vi "FormatTableStyle.vi"(7 "Format Command":T1, 8 "Error In":errorcluster, 9 "Row Index":i32, 10 "Parameter (Optional)":i32, 11 "Table reference Array":refnum<vi>[](array[refnum])) -> (0 "Error Out":errorcluster)   [LabVIEW 2012]
doc: "SciScan 1.2 160622\nThis VI implements the formatting of table data which includes highlighting, unhighlighting, and modifying visible rows (due to scrolling).\n\n<b>INPUTS</b>\n--------\n<b>Format Command </b> - Formatting action needs to be be taken\n<b>Table references array </b>- Array containing references of the tables of interest\n<b>Row </b>- Row number that needs to be fromatted"
uses:
  FormatTableStyle_Commands.ctl
  <vilib>/Utility/miscctls.llb/LVRowAndColumnTypeDef.ctl
  <vilib>/Utility/miscctls.llb/LVRowAndColumnUnsignedTypeDef.ctl
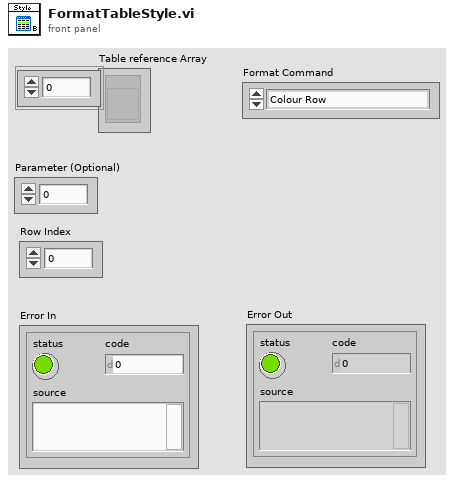
[diagram p1: front panel]
types:
  T1 = typedef "FormatTableStyle_Commands.ctl" = enum16{"Colour Row", "Uncolour Row", "Bold Row", "Clear table", "UpdateVisibleRows", "Set Row Height", "Enabled Row style", "Disabled Row Style"}
  T2 = typedef "LVRowAndColumnTypeDef.ctl" = cluster{"Row":i32, "Column":i32}
  T3 = typedef "LVRowAndColumnUnsignedTypeDef.ctl" = cluster{"Row":u32, "Column":u32}
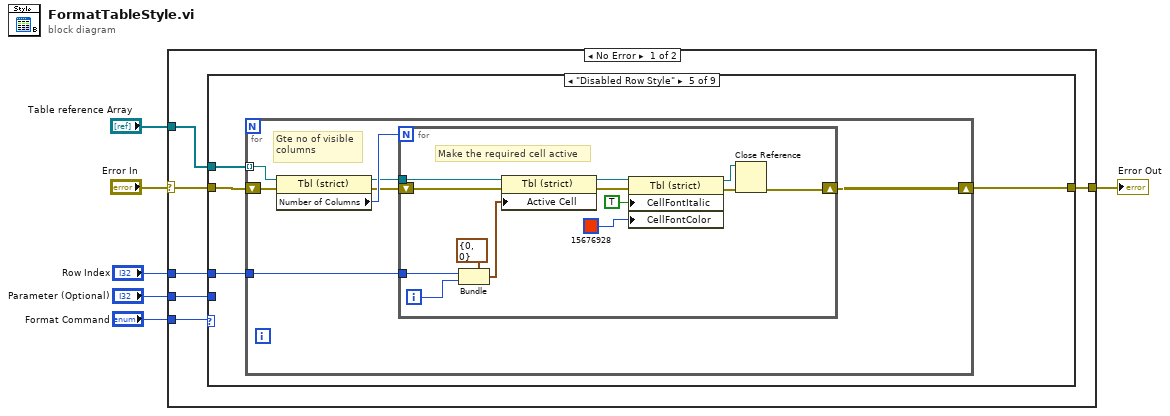
[diagram p0: block diagram]
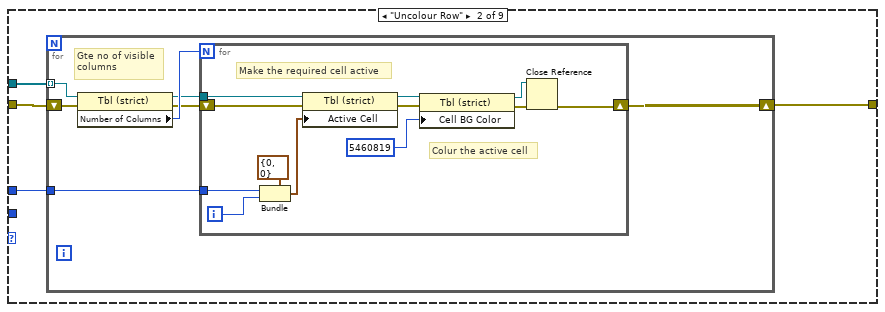
[diagram p3: hidden frame]
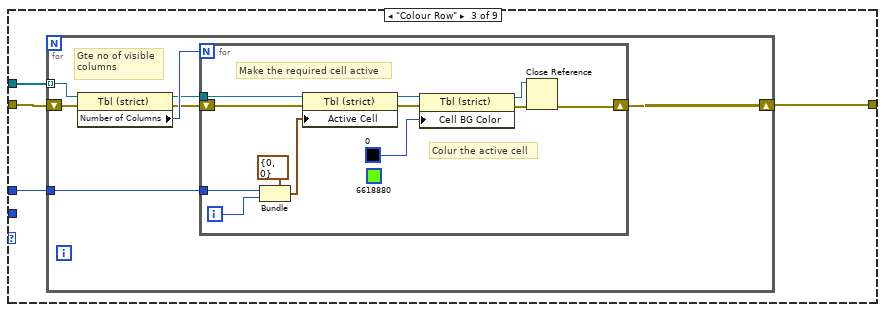
[diagram p4: hidden frame]
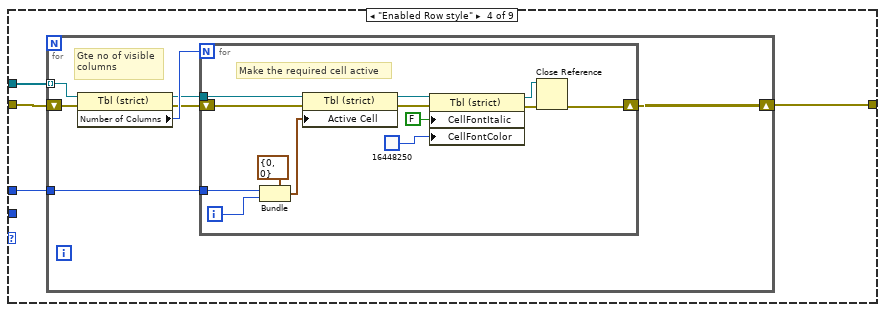
[diagram p5: hidden frame]
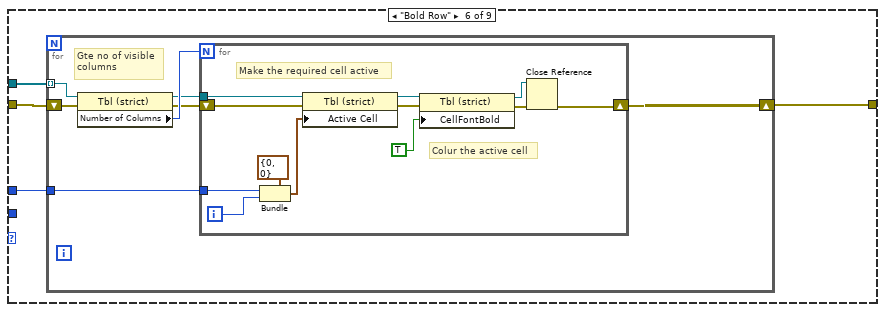
[diagram p6: hidden frame]
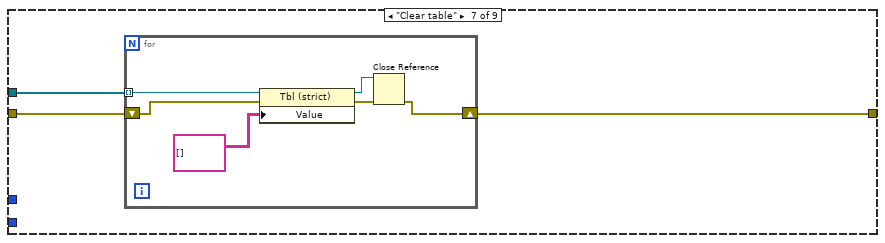
[diagram p7: hidden frame]
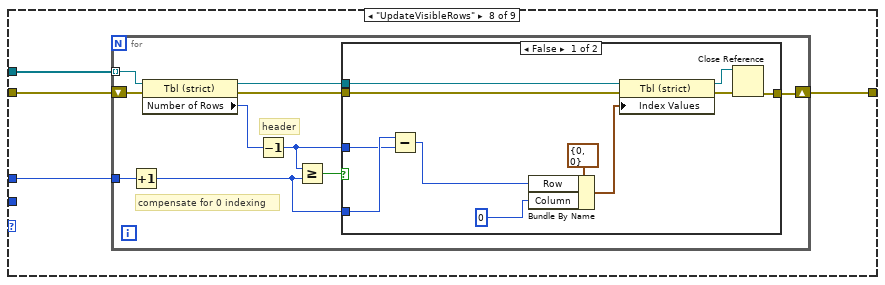
[diagram p8: hidden frame]
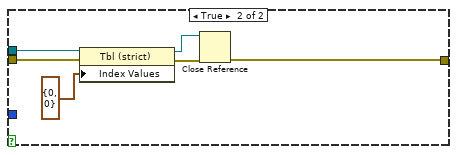
[diagram p9: hidden frame]
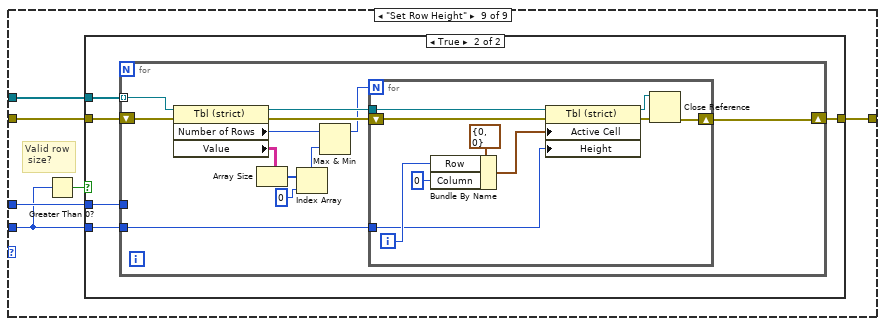
[diagram p10: hidden frame]
diagram:
  n1 = case shown="No Error" "Error In" {
    selector: "Error In" -> [w12 w205]
    tunnel: "Row Index" -> [w10 _]
    tunnel: [w9 w205] -> w4
    tunnel: "Table reference Array" -> [w11 _]
    tunnel: "Format Command" -> [w8 _]
    tunnel: "Parameter (Optional)" -> [w7 _]
    frame No Error {
      n2 = case shown="\"Disabled Row Style\"" w8 {
        tunnel: w12 -> [w13 w17 w40 w63 w87 w111 w131 w142 w175]
        tunnel: w11 -> [_ w16 w39 w62 w86 w110 w133 w143 w176]
        tunnel: w10 -> [_ w15 w38 w61 w85 w109 _ w141 w174]
        tunnel: [w13 w14 w37 w60 w84 w108 w132 w140 w173] -> w9
        tunnel: w7 -> [_ _ _ _ _ _ _ _ w171]
        frame Default {
        }
        frame "Uncolour Row" {
          n3 = for {
            tunnel: w15 -> [w22]
            tunnel: w16 -> [w24] mode=indexing
            shift-right: [w18] -> w14
            shift-left: w17 -> [w21]
            # "Gte no of visible\ncolumns"
            n4 = property class="Tbl (strict)"(reference=w24, error in=w21) -> (reference out=w20:refnum<vi>, error out=w19:errorcluster, "Number of Columns"=w23:u32)
            n5 = for {
              N: w23 -> [_]
              tunnel: w22 -> [w26]
              tunnel: w20 -> [w32]
              shift-right: [w30] -> w18
              shift-left: w19 -> [w31]
              i -> [w27]
              # "Colur the active cell"
              # "Make the required cell active"
              n6 = Bundle(cluster=T2 {"Row"=0, "Column"=0} ("Active Cell:Active Cell"), "Row"=w26, "Column"=w27) -> (w28:T2)
              n7 = property class="Tbl (strict)"(reference=w32, error in=w31, "Active Cell"=w28) -> (reference out=w36:refnum<vi>, error out=w35:errorcluster)
              n8 = property class="Tbl (strict)"(reference=w36, error in=w35, "Cell BG Color"=u32 5460819 ("Active Cell:Cell Background Color")) -> (reference out=w33:refnum<vi>, error out=w34:errorcluster)
              n9 = Close Reference(reference=w33, error in (no error)=w34) -> (error out=w30:errorcluster)
            }
          }
        }
        frame "Colour Row" {
          n10 = for {
            tunnel: w38 -> [w45]
            tunnel: w39 -> [w47] mode=indexing
            shift-right: [w41] -> w37
            shift-left: w40 -> [w44]
            # "Gte no of visible\ncolumns"
            n11 = property class="Tbl (strict)"(reference=w47, error in=w44) -> (reference out=w43:refnum<vi>, error out=w42:errorcluster, "Number of Columns"=w46:u32)
            n12 = for {
              N: w46 -> [_]
              tunnel: w45 -> [w49]
              tunnel: w43 -> [w55]
              shift-right: [w53] -> w41
              shift-left: w42 -> [w54]
              i -> [w50]
              (unwired) u32 6618880 ("Background colour")
              # "Colur the active cell"
              # "Make the required cell active"
              n13 = Bundle(cluster=T2 {"Row"=0, "Column"=0} ("Active Cell:Active Cell"), "Row"=w49, "Column"=w50) -> (w51:T2)
              n14 = property class="Tbl (strict)"(reference=w55, error in=w54, "Active Cell"=w51) -> (reference out=w59:refnum<vi>, error out=w58:errorcluster)
              n15 = property class="Tbl (strict)"(reference=w59, error in=w58, "Cell BG Color"=u32 0 ("Background colour")) -> (reference out=w56:refnum<vi>, error out=w57:errorcluster)
              n16 = Close Reference(reference=w56, error in (no error)=w57) -> (error out=w53:errorcluster)
            }
          }
        }
        frame "Enabled Row style" {
          n17 = for {
            tunnel: w61 -> [w68]
            tunnel: w62 -> [w70] mode=indexing
            shift-right: [w64] -> w60
            shift-left: w63 -> [w67]
            # "Gte no of visible\ncolumns"
            n18 = property class="Tbl (strict)"(reference=w70, error in=w67) -> (reference out=w66:refnum<vi>, error out=w65:errorcluster, "Number of Columns"=w69:u32)
            n19 = for {
              N: w69 -> [_]
              tunnel: w68 -> [w73]
              tunnel: w66 -> [w79]
              shift-right: [w77] -> w64
              shift-left: w65 -> [w78]
              i -> [w74]
              # "Make the required cell active"
              n20 = Bundle(cluster=T2 {"Row"=0, "Column"=0} ("Active Cell:Active Cell"), "Row"=w73, "Column"=w74) -> (w75:T2)
              n21 = property class="Tbl (strict)"(reference=w79, error in=w78, "Active Cell"=w75) -> (reference out=w83:refnum<vi>, error out=w82:errorcluster)
              n22 = property class="Tbl (strict)"(reference=w83, error in=w82, "CellFontItalic"=FALSE ("Active Cell:Cell Font:Italic"), "CellFontColor"=u32 16448250 ("Background colour")) -> (reference out=w80:refnum<vi>, error out=w81:errorcluster)
              n23 = Close Reference(reference=w80, error in (no error)=w81) -> (error out=w77:errorcluster)
            }
          }
        }
        frame "Disabled Row Style" {
          n24 = for {
            tunnel: w85 -> [w92]
            tunnel: w86 -> [w94] mode=indexing
            shift-right: [w88] -> w84
            shift-left: w87 -> [w91]
            # "Gte no of visible\ncolumns"
            n25 = property class="Tbl (strict)"(reference=w94, error in=w91) -> (reference out=w90:refnum<vi>, error out=w89:errorcluster, "Number of Columns"=w93:u32)
            n26 = for {
              N: w93 -> [_]
              tunnel: w92 -> [w97]
              tunnel: w90 -> [w103]
              shift-right: [w101] -> w88
              shift-left: w89 -> [w102]
              i -> [w98]
              # "Make the required cell active"
              n27 = Bundle(cluster=T2 {"Row"=0, "Column"=0} ("Active Cell:Active Cell"), "Row"=w97, "Column"=w98) -> (w99:T2)
              n28 = property class="Tbl (strict)"(reference=w103, error in=w102, "Active Cell"=w99) -> (reference out=w107:refnum<vi>, error out=w106:errorcluster)
              n29 = property class="Tbl (strict)"(reference=w107, error in=w106, "CellFontItalic"=TRUE ("Active Cell:Cell Font:Italic"), "CellFontColor"=u32 15676928 ("Background colour")) -> (reference out=w104:refnum<vi>, error out=w105:errorcluster)
              n30 = Close Reference(reference=w104, error in (no error)=w105) -> (error out=w101:errorcluster)
            }
          }
        }
        frame "Bold Row" {
          n31 = for {
            tunnel: w109 -> [w116]
            tunnel: w110 -> [w118] mode=indexing
            shift-right: [w112] -> w108
            shift-left: w111 -> [w115]
            # "Gte no of visible\ncolumns"
            n32 = property class="Tbl (strict)"(reference=w118, error in=w115) -> (reference out=w114:refnum<vi>, error out=w113:errorcluster, "Number of Columns"=w117:u32)
            n33 = for {
              N: w117 -> [_]
              tunnel: w116 -> [w120]
              tunnel: w114 -> [w126]
              shift-right: [w124] -> w112
              shift-left: w113 -> [w125]
              i -> [w121]
              # "Colur the active cell"
              # "Make the required cell active"
              n34 = Bundle(cluster=T2 {"Row"=0, "Column"=0} ("Active Cell:Active Cell"), "Row"=w120, "Column"=w121) -> (w122:T2)
              n35 = property class="Tbl (strict)"(reference=w126, error in=w125, "Active Cell"=w122) -> (reference out=w130:refnum<vi>, error out=w129:errorcluster)
              n36 = property class="Tbl (strict)"(reference=w130, error in=w129, "CellFontBold"=TRUE ("Active Cell:Cell Font:Bold")) -> (reference out=w127:refnum<vi>, error out=w128:errorcluster)
              n37 = Close Reference(reference=w127, error in (no error)=w128) -> (error out=w124:errorcluster)
            }
          }
        }
        frame "Clear table" {
          n38 = for {
            tunnel: w133 -> [w138] mode=indexing
            shift-right: [w136] -> w132
            shift-left: w131 -> [w134]
            n39 = property class="Tbl (strict)"(reference=w138, error in=w134, "Value"=string[][] []) -> (reference out=w135:refnum<vi>, error out=w139:errorcluster)
            n40 = Close Reference(reference=w135, error in (no error)=w139) -> (error out=w136:errorcluster)
          }
        }
        frame "UpdateVisibleRows" {
          n41 = for {
            tunnel: w143 -> [w153] mode=indexing
            shift-right: [w147] -> w140
            shift-left: w142 -> [w152]
            tunnel: w141 -> [w151]
            # "compensate for 0 indexing"
            # "header"
            n42 = Increment(x=w151) -> (x+1=w146:i32)
            n43 = property class="Tbl (strict)"(reference=w153, error in=w152) -> (reference out=w148:refnum<vi>, error out=w149:errorcluster, "Number of Rows"=w145:u32)
            n44 = Decrement(x=w145) -> (x-1=w144:u32)
            n45 = Greater Or Equal?(x=w144, y=w146) -> (x >= y?=w150:bool)
            n46 = case shown="False" w150 {
              tunnel: w149 -> [w163 w169]
              tunnel: w148 -> [w164 w170]
              tunnel: [w161 w166] -> w147
              tunnel: w144 -> [w155 _]
              tunnel: w146 -> [w156 _]
              frame False {
                n47 = Subtract(x=w156, y=w155) -> (x-y=w154:u32)
                n48 = Bundle By Name(cluster=T3 {"Row"=0, "Column"=0} ("Index Values"), "Row"=w154, "Column"=u32 0) -> (w157:T3)
                n49 = property class="Tbl (strict)"(reference=w164, error in=w163, "Index Values"=w157) -> (reference out=w159:refnum<vi>, error out=w160:errorcluster)
                n50 = Close Reference(reference=w159, error in (no error)=w160) -> (error out=w161:errorcluster)
              }
              frame True {
                n51 = property class="Tbl (strict)"(reference=w170, error in=w169, "Index Values"=T3 {"Row"=0, "Column"=0}) -> (reference out=w165:refnum<vi>, error out=w167:errorcluster)
                n52 = Close Reference(reference=w165, error in (no error)=w167) -> (error out=w166:errorcluster)
              }
            }
          }
        }
        frame "Set Row Height" {
          # "Valid row\n size?"
          n53 = Greater Than 0?(x=w171) -> (x > 0?=w172:bool)
          n54 = case shown="True" w172 {
            tunnel: w176 -> [_ w182]
            tunnel: w175 -> [w177 w181]
            tunnel: w174 -> [_ w180]
            tunnel: [w177 w179] -> w173
            tunnel: w171 -> [_ w178]
            frame False {
            }
            frame True {
              n55 = for {
                tunnel: w182 -> [w194] mode=indexing
                shift-right: [w190] -> w179
                shift-left: w181 -> [w193]
                tunnel: w180 -> [_]
                tunnel: w178 -> [w183]
                n56 = property class="Tbl (strict)"(reference=w194, error in=w193) -> (reference out=w191:refnum<vi>, error out=w192:errorcluster, "Number of Rows"=w189:u32, "Value"=w188:string[][])
                n57 = Array Size(array=w188) -> (size(s)=w187:i32[])
                n58 = Index Array(array=w187, index=0) -> (element=w185:i32)
                n59 = Max & Min(x=w189, y=w185) -> (max(x,y)=w184:u32)  [unwired: 1 out]
                n60 = for {
                  N: w184 -> [_]
                  tunnel: w191 -> [w203]
                  shift-right: [w202] -> w190
                  shift-left: w192 -> [w204]
                  tunnel: w183 -> [w195]
                  i -> [w197]
                  n61 = Bundle By Name(cluster=T3 {"Row"=0, "Column"=0} ("Index Values"), "Row"=w197, "Column"=u32 0) -> (w198:T3)
                  n62 = property class="Tbl (strict)"(reference=w203, error in=w204, "Active Cell"=w198, "Height"=w195) -> (reference out=w196:refnum<vi>, error out=w200:errorcluster)
                  n63 = Close Reference(reference=w196, error in (no error)=w200) -> (error out=w202:errorcluster)
                }
              }
            }
          }
        }
      }
    }
    frame Error {
    }
  }
  "Error Out" <- w4
